vi "Noise (G3)-Compute Max Level.vi"(0 "Noise Params":T6, 5 "Filter":T3 {"Stages"."IIR Filter"."Forward Coefficients" format="%.4f"; "Stages"."IIR Filter"."Reverse Coefficients" format="%.4f"}, 9 "Level":T1, 11 "error in (no error)":errorcluster, 12 "Sampling Rate (Hz)":dbl, 13 "Npts":i32) -> (6 "Max Level":dbl, 10 "Level out":T1, 15 "error out":errorcluster)   [LabVIEW 2020]
uses:
  Noise (G3).ctl
  Noise (G3).Properties.ctl
  Noise (G3).Data.ctl
  XControls/Filter (G3)/Filter Data.ctl
  XControls/Filter (G3)/Filter Type.ctl
  Filter VIs/Filter-Bandwidth Units.ctl
  XControls/Level (G3)/Level Data.ctl
  XControls/Level (G3)/Level Units (G3).ctl
  <vilib>/Analysis/5stat.llb/RMS (DBL).vi
  Waveform VIs/Noise VIs/Noise-Globals.vi
  PXI DAQ VIs/DAQ Engine VIs/PXI Globals.vi
  Utility VIs/Math VIs/Linear to dB (scalar).vi
  <vilib>/Analysis/NI_AALPro.lvlib
  4th Generation/Classes/Filter/Filter.lvclass
  XControls/Level (G3)/Level (G3).xctl
  XControls/Filter (G3)/Filter (G3).xctl
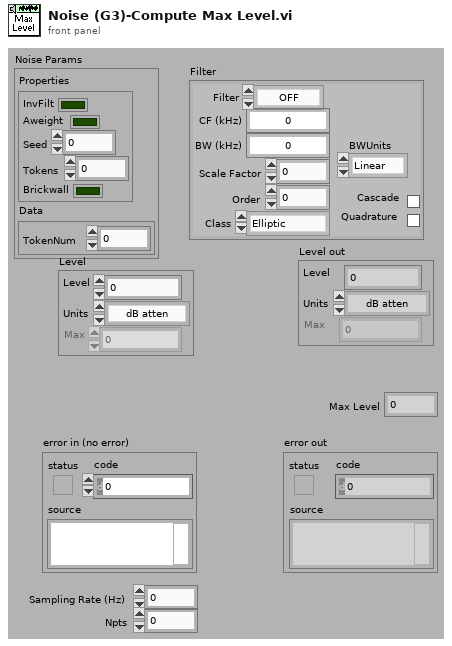
[diagram p1: front panel]
types:
  T1 = typedef "Level (G3).xctl/Level Data.ctl" = cluster{"Level":dbl, "Units":T2, "Max":dbl, "Data":cluster{"Multiplier":dbl, "Cal File":path, "Cal":cluster{"Freq (Hz)":dbl[], "Mag (dB SPL)":dbl[], "Phase (deg)":dbl[]}, "audiogram":path}}
  T2 = typedef "Level (G3).xctl/Level Units (G3).ctl" = enum16{"dB atten", "dB SPL", "dB re 1 Vrms", "dB V/Hz½", "mW", "dB HL", "Volts", "dB mW"}
  T3 = typedef "Filter (G3).xctl/Filter Data.ctl" = cluster{"Type":T4, "CF (kHz)":dbl, "BW (kHz)":dbl, "Cascade":bool, "Quadrature":bool, "Scale Factor":dbl, "Stages":cluster{"IIR Filter":cluster{"filter structure":enum32{"IIR 2nd Order", "IIR 4th Order"}, "Reverse Coefficients":dbl[], "Forward Coefficients":dbl[]}, "State":dbl[]}[], "Class":enum16{"Elliptic", "Butterworth"}, "Order":i32, "BWUnits":T5}
  T4 = typedef "Filter (G3).xctl/Filter Type.ctl" = enum16{"OFF", "Lowpass", "Highpass", "Bandpass", "Bandstop"}
  T5 = typedef "Filter-Bandwidth Units.ctl" = enum16{"Linear", "Octaves", "Min-Max"}
  T6 = typedef "Noise (G3).ctl" = cluster{"Properties":T7, "Data":T8}
  T7 = typedef "Noise (G3).Properties.ctl" = cluster{"InvFilt":bool, "Aweight":bool, "Seed":i32, "Tokens":i32, "Brickwall":bool}
  T8 = typedef "Noise (G3).Data.ctl" = cluster{"TokenNum":i32}
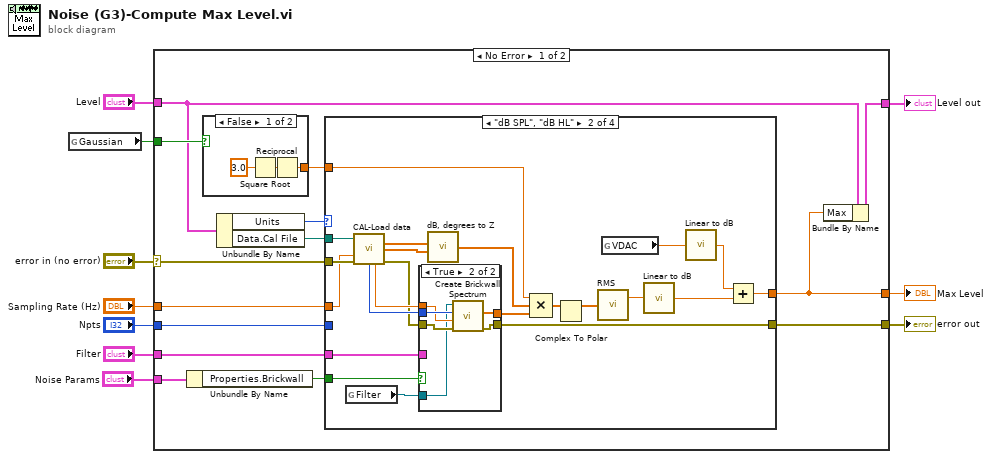
[diagram p0: block diagram]
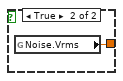
[diagram p2: hidden frame]
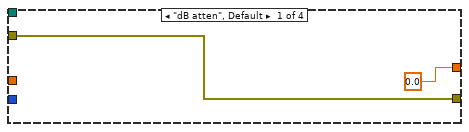
[diagram p3: hidden frame]
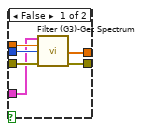
[diagram p4: hidden frame]
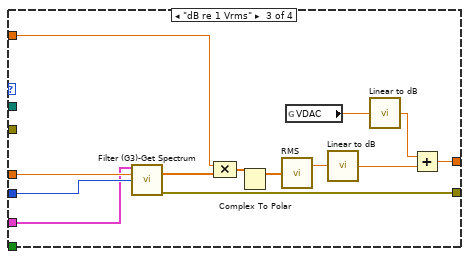
[diagram p5: hidden frame]
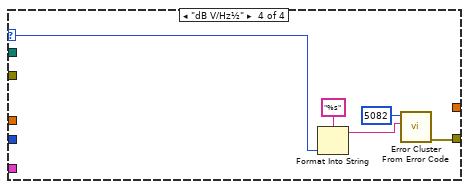
[diagram p6: hidden frame]
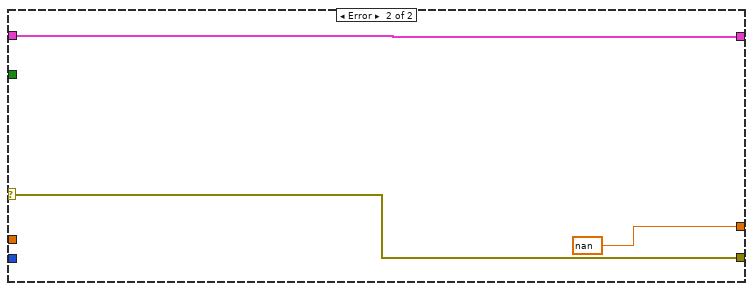
[diagram p7: hidden frame]
diagram:
  n1 = global read "Noise-Globals.vi" "Gaussian"() -> (w1:bool)
  n2 = case shown="No Error" "error in (no error)" {
    selector: "error in (no error)" -> [w24 w85]
    tunnel: "Level" -> [w13 w83]
    tunnel: "Noise Params" -> [w12 _]
    tunnel: "Filter" -> [w22 _]
    tunnel: [w20 w85] -> w9
    tunnel: "Npts" -> [w23 _]
    tunnel: [w19 nan ("Reference Level")] -> w4
    tunnel: "Sampling Rate (Hz)" -> [w21 _]
    tunnel: [w18 w83] -> w2
    tunnel: w1 -> [w15 _]
    frame No Error {
      n3 = Unbundle By Name(w12) -> ("Properties.Brickwall"=w11:bool)
      n4 = case shown="False" w15 {
        tunnel: [w27 w28] -> w16
        frame False {
          n5 = Square Root(x=3.0 ("Noise Vrms")) -> (sqrt(x)=w25:dbl)
          n6 = Reciprocal(x=w25) -> (1/x=w27:dbl)
        }
        frame True {
          n7 = global read "Noise-Globals.vi" "Noise.Vrms"() -> (w28:dbl)
        }
      }
      n8 = Unbundle By Name(w13) -> ("Units"=w17:T2, "Data.Cal File"=w14:path)
      n9 = case shown="\"dB SPL\", \"dB HL\"" w17 {
        selector: w17 -> [_ _ _ w78]
        tunnel: w24 -> [w29 w52 _ _]
        tunnel: w23 -> [_ _ w67 _]
        tunnel: w22 -> [_ w34 w65 _]
        tunnel: [0.0 ("Reference Level") w47 w76 _] -> w19
        tunnel: w21 -> [_ w33 w68 _]
        tunnel: [w29 w36 w69 w79] -> w20
        tunnel: w14 -> [_ w45 _ _]
        tunnel: w16 -> [_ w35 w66 _]
        tunnel: w11 -> [_ w32 _ _]
        frame "dB atten", Default {
        }
        frame "dB SPL", "dB HL" {
          n10 = global read "Noise-Globals.vi" "Filter"() -> (w31:refnum<class "Filter.lvclass">)
          n11 = call "CAL-Load data.vi"("user path"=w45, "Desired Fs (Hz)"=w33, "error in (no error)"=w52) -> ("Mag"=w44:dbl[], "Phase"=w43:dbl[], "npts"=w50:i32, "Fs (Hz)"=w51:dbl, "error out"=w49:errorcluster)  [unwired: 5 in, 3 out]
          n12 = case shown="True" w32 {
            tunnel: w51 -> [w58 w63]
            tunnel: w50 -> [w57 w64]
            tunnel: w49 -> [w56 w60]
            tunnel: [w55 w62] -> w40
            tunnel: [w54 w61] -> w36
            tunnel: w34 -> [w53 _]
            tunnel: w31 -> [_ w59]
            frame False {
              n13 = call "Filter (G3)-Get Spectrum.vi"("Filter in"=w53, "Sampling Rate (Hz)"=w58, "Npts"=w57, "error in (no error)"=w56) -> ("spectrum"=w55:cdb[], "error out"=w54:errorcluster)  [unwired: 9 in, 1 out]
            }
            frame True {
              n14 = call "Create Brickwall Spectrum.vi"("error in (no error)"=w60, "Fs (Hz)"=w63, "Npts"=w64, "Filter in"=w59) -> ("error out"=w61:errorcluster, "Spectrum"=w62:dbl[])  [unwired: 5 in, 1 out]
            }
          }
          n15 = call "dB, degrees to Z.vi"("Magnitude (dB)"=w44, "Phase (degrees)"=w43) -> ("Z"=w39:cdb[])  [unwired: 5 in]
          n16 = Compound Arithmetic op=MULTIPLY(w35, w39, w40) -> (w41:cdb[])
          n17 = Complex To Polar(r * e^(i*theta)=w41) -> (r=w38:dbl[])  [unwired: 1 out]
          n18 = call-poly <vilib>:"RMS.vi"("X"=w38) -> ("rms value"=w42:dbl)  [unwired: 1 out]
          n19 = global read "PXI Globals.vi" "VDAC"() -> (w48:dbl)
          n20 = call-poly "Linear to dB.vi"("Linear"=w42) -> ("dB"=w37:dbl)
          n21 = call-poly "Linear to dB.vi"("Linear"=w48) -> ("dB"=w46:dbl)
          n22 = Add(x=w46, y=w37) -> (x+y=w47:dbl)
        }
        frame "dB re 1 Vrms" {
          n23 = call "Filter (G3)-Get Spectrum.vi"("Filter in"=w65, "Sampling Rate (Hz)"=w68, "Npts"=w67) -> ("spectrum"=w72:cdb[], "error out"=w69:errorcluster)  [unwired: 10 in, 1 out]
          n24 = Compound Arithmetic op=MULTIPLY(w66, w72) -> (w73:cdb[])
          n25 = Complex To Polar(r * e^(i*theta)=w73) -> (r=w71:dbl[])  [unwired: 1 out]
          n26 = call-poly <vilib>:"RMS.vi"("X"=w71) -> ("rms value"=w74:dbl)  [unwired: 1 out]
          n27 = global read "PXI Globals.vi" "VDAC"() -> (w77:dbl)
          n28 = call-poly "Linear to dB.vi"("Linear"=w74) -> ("dB"=w70:dbl)
          n29 = call-poly "Linear to dB.vi"("Linear"=w77) -> ("dB"=w75:dbl)
          n30 = Add(x=w75, y=w70) -> (x+y=w76:dbl)
        }
        frame "dB V/Hz½" {
          n31 = Format Into String(format string="%s", w78) -> (resulting string=w81:string)  [unwired: 2 in, 1 out]
          n32 = call <vilib>:"Error Cluster From Error Code.vi"("error message (\"\")"=w81, "error code (0)"=5082) -> ("error out"=w79:errorcluster)  [unwired: 7 in]
        }
      }
      n33 = Bundle By Name(cluster=w13, "Max"=w19) -> (w18:T1)
    }
    frame Error {
    }
  }
  "error out" <- w9
  "Max Level" <- w4
  "Level out" <- w2
